vi "AMB_Dual_Interface_Close.vi"(1 "Error In":errorcluster {"code" format="%.0x"}, 2 "Object\nHandle":u32) -> (0 "Error Out":errorcluster {"code" format="%.0x"})   [LabVIEW 2017]
doc: "This VI close the communication with a CAN node or an open TCP/IP port.\nIt uses the global variable 'AMB_Global.gbl.vi' to determine if communication is done directly with a CAN interface or if the CAN commands are tunneled through TCP/IP."
uses:
  AMB_Global.gbl.vi
panel:
  in  "TCP Connection ID":refnum<k5>
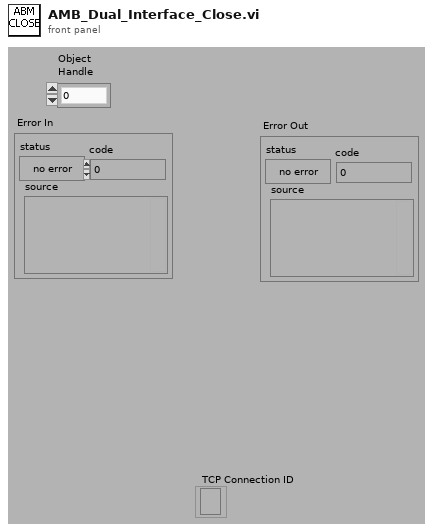
[diagram p1: front panel]
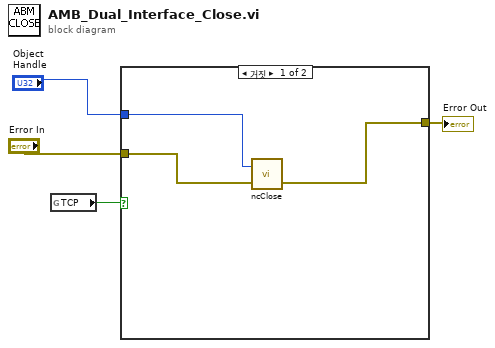
[diagram p0: block diagram]
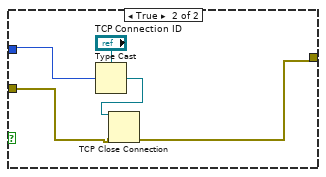
[diagram p2: hidden frame]
diagram:
  n1 = global read "AMB_Global.gbl.vi" "TCP"() -> (w4:bool)
  n2 = case shown="거짓" w4 {
    tunnel: "Error In" -> [w7 w12]
    tunnel: "Object\nHandle" -> [w6 w8]
    tunnel: [w5 w11] -> w1
    frame False {
      n3 = call <vilib>:"ncClose.vi"("Error in"=w7, "ObjHandle in"=w6) -> ("Error out"=w5:errorcluster)  [unwired: 1 in]
    }
    frame True {
      n4 = Type Cast(type="TCP Connection ID", x=w8) -> (*(type *) &x=w9:refnum<k5>)
      n5 = TCP Close Connection(connection ID=w9, error in (no error)=w12) -> (error out=w11:errorcluster)  [unwired: 1 in, 1 out]
    }
  }
  "Error Out" <- w1
